vi "Analog Output (FPGA).vi"() -> ()   [LabVIEW 2011]
doc: "This VI will continually write single point values to 4 channels of an analog output module."
uses:
  <vilib>/rvi/eio/common/nirviEmuTemplateMethod_errors.vi
  <vilib>/eio/EIONode/EIONode.xnode
panel:
  in  "stop":bool
  in  "AO Data":T1
  out "FPGA Error Out":errorcluster
  # "For instructions, and select Help>>Show Context Help and hover over the icon."
  # "Input Parameters"
  # "Output Parameters"
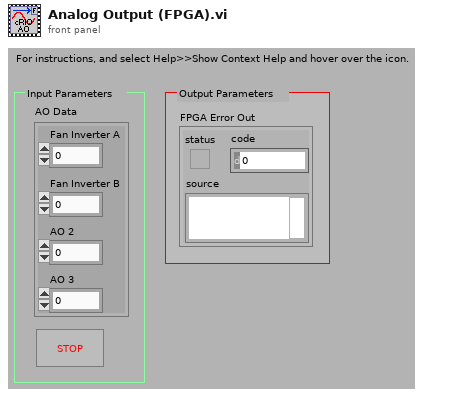
[diagram p1: front panel]
types:
  T1 = cluster{"Fan Inverter A":fxp<+/-,20,5>, "Fan Inverter B":fxp<+/-,20,5>, "AO 2":fxp<+/-,20,5>, "AO 3":fxp<+/-,20,5>}
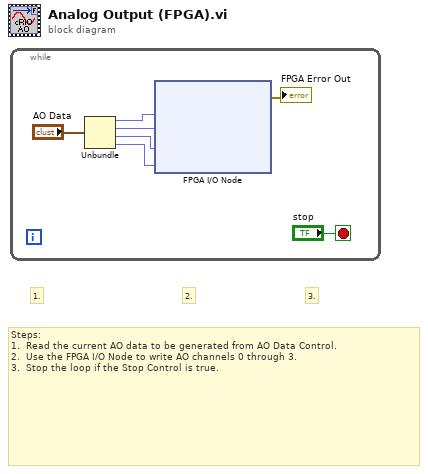
[diagram p0: block diagram]
diagram:
  # "3."
  # "2."
  # "1."
  # "Steps: \n1.  Read the current AO data to be generated from AO Data Control.\n2.  Use the FPGA I/O Node to write AO channels 0 through 3. \n3.  Stop the loop if the Stop Control is true."
  n1 = while {
    stop <- "stop" stop-if-true
    n2 = Unbundle("AO Data") -> ("Fan Inverter A"=w4:fxp<+/-,20,5>, "Fan Inverter B"=w3:fxp<+/-,20,5>, "AO 2"=w2:fxp<+/-,20,5>, "AO 3"=w1:fxp<+/-,20,5>)
    n3 = xnode "FPGA I/O Node"("Inverter Fan A"=w4, "Inverter Fan B"=w3, "Mod5/AO2"=w2, "Mod5/AO3"=w1) -> ("error out"=→"FPGA Error Out":errorcluster)  [unwired: 5 in, 4 out]
  }
